vi "Keithley 6514 Buffer Read.vi"(0 "Resource In":refnum<visa-resource-name>, 1 "Check For SCPI Errors? (T)":bool=TRUE, 11 "error in (no error)":T1) -> (4 "Resource Out (dupl)":refnum<visa-resource-name>, 6 "Num Readings":i32 min=0 max=2500, 8 "Test Data":sgl[][](array[numeric]) format="%^.4e", 10 "Data Elements":string, 15 "error out":T1)   [LabVIEW 2009, in "Keithley 6514 LV 2009.lvlib"]
doc: "This VI is used to retrieve data from the Instrument's data buffer. The VI will return the number of points that was stored in the buffer, the data format used for the data transfer, the data elements returned and the actual data which is stored in a LabVIEW array.\n\nDEFAULTS: \nGPIB Address = 7\n\nPoints Stored in Buffer:\nReturned by Instrument. Not user settable. 2 to 1024.\n\nData Format: \nReturned by Instrument. Not user settable. Format returned is 'ASC' for ASCII and 'SRE' for Single Precision Real.\n\nData Elements:\nReturned by Instrument. Not user settable. The order in which the elements are returned reflects the order in which each data point is presented in the array. Main order is:\nReading, Channel Number\n\nTest Data:\nThis is an array where the buffer data is placed after transfer over the bus. The order for which the data is presented appears in the 'Data Elements' indicator. Maximum number of data points returned is 1024."
uses:
  Keithley 6514 LV 2009.lvlib
panel:
  in  "Timeout (5000 msecs)":u32=5000
  out "Num Bytes To Read For Binary":i32
  out "Data Format":string
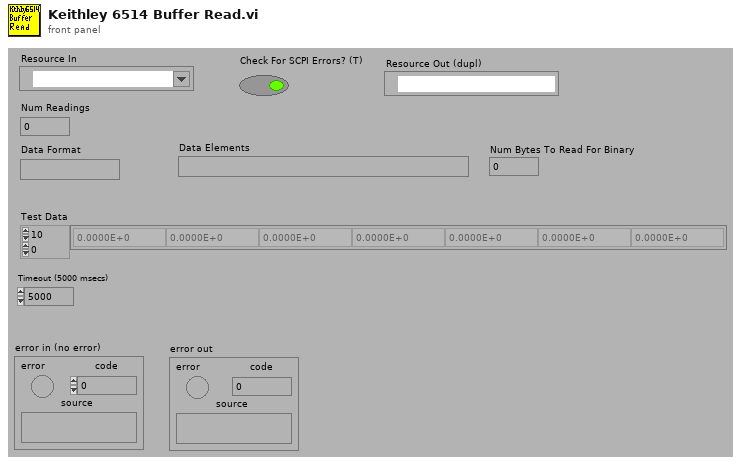
[diagram p1: front panel]
types:
  T1 = cluster{"error":bool, "code":i32, "source":string}
  T2 = enum16{"big-endian, network order", "native, host order", "little-endian"}
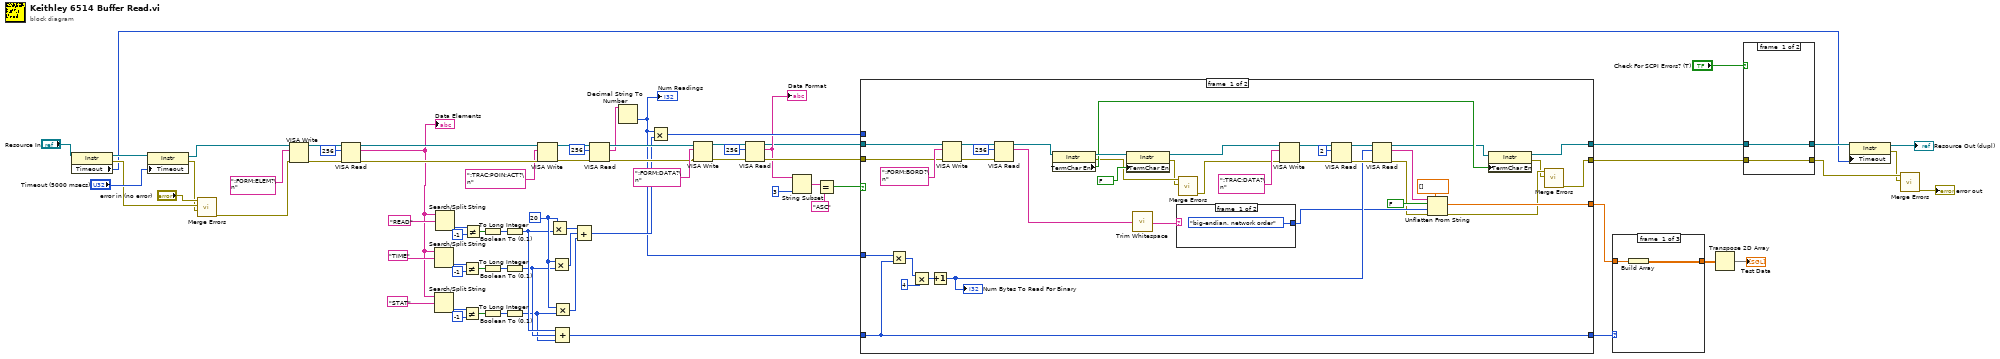
[diagram p0: block diagram]
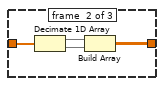
[diagram p2: hidden frame]
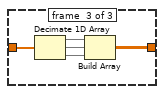
[diagram p3: hidden frame]
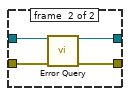
[diagram p4: hidden frame]
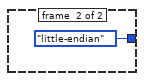
[diagram p5: hidden frame]
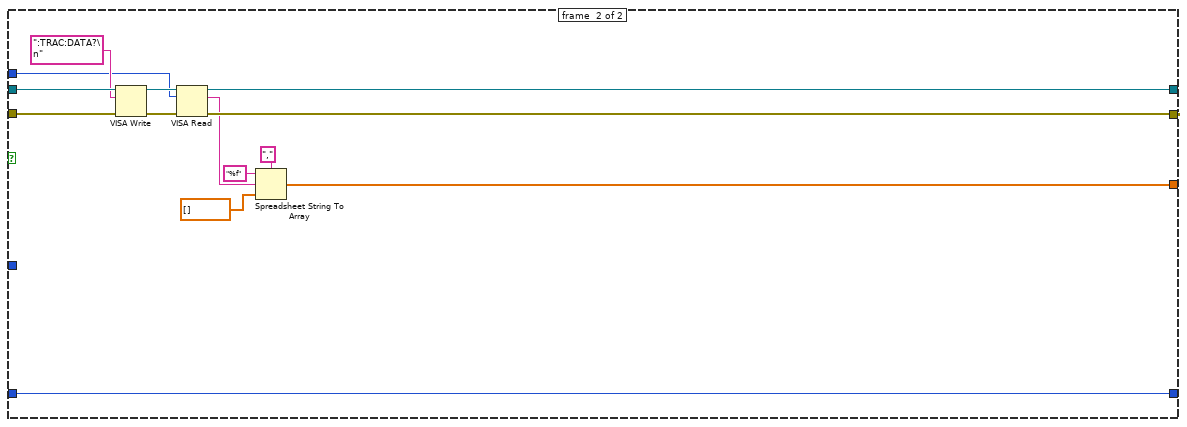
[diagram p6: hidden frame]
diagram:
  w28 = 20 ("x")
  n1 = property class="Instr"(reference="Resource In") -> (reference out=w12:refnum<visa-resource-name>, error out=w10:errorcluster, "Timeout"=w4:u32)  [unwired: 1 in]
  n2 = property class="Instr"(reference=w12, "Timeout"="Timeout (5000 msecs)") -> (reference out=w7:refnum<visa-resource-name>, error out=w9:errorcluster)  [unwired: 1 in]
  n3 = call <vilib>:"Merge Errors.vi"("error in 3 (no error)"=w9, "error in 2 (no error)"=w10, "error in 1 (no error)"="error in (no error)") -> ("error out"=w8:errorcluster)  [unwired: 4 in]
  n4 = VISA Write(VISA resource name=w7, write buffer=":FORM:ELEM?\n", error in (no error)=w8) -> (VISA resource name out=w65:refnum<visa-resource-name>, error out=w64:errorcluster)  [unwired: 1 out]
  n5 = VISA Read(VISA resource name=w65, byte count=u32 256, error in (no error)=w64) -> (VISA resource name out=w58:refnum<visa-resource-name>, read buffer=w36:string, error out=w59:errorcluster)  [unwired: 1 out]
  "Data Elements" <- w36
  n6 = Search/Split String(string=w36, search string/char (-)="TIME") -> (offset of match=w41:i32)  [unwired: 1 in, 2 out]
  n7 = Search/Split String(string=w36, search string/char (-)="STAT") -> (offset of match=w38:i32)  [unwired: 1 in, 2 out]
  n8 = Search/Split String(string=w36, search string/char (-)="READ") -> (offset of match=w43:i32)  [unwired: 1 in, 2 out]
  n9 = Not Equal?(x=w41, y=-1) -> (x != y?=w33:bool)
  n10 = Not Equal?(x=w38, y=-1) -> (x != y?=w32:bool)
  n11 = Not Equal?(x=w43, y=-1) -> (x != y?=w34:bool)
  n12 = Boolean To (0,1)(Boolean=w34) -> (0, 1=w31:i16)
  n13 = Boolean To (0,1)(Boolean=w33) -> (0, 1=w30:i16)
  n14 = Boolean To (0,1)(Boolean=w32) -> (0, 1=w29:i16)
  n15 = To Long Integer(number=w31) -> (32bit integer=w23:i32)
  n16 = To Long Integer(number=w30) -> (32bit integer=w22:i32)
  n17 = To Long Integer(number=w29) -> (32bit integer=w21:i32)
  n18 = VISA Write(VISA resource name=w58, write buffer=":TRAC:POIN:ACT?\n", error in (no error)=w59) -> (VISA resource name out=w61:refnum<visa-resource-name>, error out=w60:errorcluster)  [unwired: 1 out]
  n19 = Multiply(x=w28, y=w23) -> (x*y=w27:i32)
  n20 = Multiply(x=w28, y=w22) -> (x*y=w26:i32)
  n21 = Multiply(x=w28, y=w21) -> (x*y=w25:i32)
  n22 = Compound Arithmetic op=ADD(w23, w22, w21) -> (w20:i32)
  n23 = Compound Arithmetic op=ADD(w27, w26, w25) -> (w24:i32)
  n24 = VISA Read(VISA resource name=w61, byte count=u32 256, error in (no error)=w60) -> (VISA resource name out=w52:refnum<visa-resource-name>, read buffer=w50:string, error out=w51:errorcluster)  [unwired: 1 out]
  n25 = Decimal String To Number(string=w50) -> (number=w19:i32)  [unwired: 2 in, 1 out]
  "Num Readings" <- w19
  n26 = Multiply(x=w19, y=w24) -> (x*y=w68:i32)
  n27 = VISA Write(VISA resource name=w52, write buffer=":FORM:DATA?\n", error in (no error)=w51) -> (VISA resource name out=w55:refnum<visa-resource-name>, error out=w54:errorcluster)  [unwired: 1 out]
  n28 = VISA Read(VISA resource name=w55, byte count=u32 256, error in (no error)=w54) -> (VISA resource name out=w47:refnum<visa-resource-name>, read buffer=w48:string, error out=w49:errorcluster)  [unwired: 1 out]
  "Data Format" <- w48
  n29 = String Subset(string=w48, length (rest)=3) -> (substring=w70:string)  [unwired: 1 in]
  n30 = Equal?(x=w70, y="ASC") -> (x = y?=w69:bool)
  n31 = case shown="False" w69 {
    tunnel: w49 -> [w90 w126]
    tunnel: w68 -> [_ w120]
    tunnel: w20 -> [w79 w114]
    tunnel: w19 -> [w109 _]
    tunnel: [w73 w127] -> w44
    tunnel: w47 -> [w91 w125]
    tunnel: [w96 w121] -> w45
    tunnel: [w80 w115] -> w17
    tunnel: [w79 w114] -> w18
    frame #0 {
      n32 = Multiply(x=w109, y=w79) -> (x*y=w111:i32)
      n33 = Multiply(x=w111, y=4) -> (x*y=w108:i32)
      n34 = Increment(x=w108) -> (x+1=w89:i32)
      "Num Bytes To Read For Binary" <- w89
      n35 = VISA Write(VISA resource name=w91, write buffer=":FORM:BORD?\n", error in (no error)=w90) -> (VISA resource name out=w94:refnum<visa-resource-name>, error out=w93:errorcluster)  [unwired: 1 out]
      n36 = VISA Read(VISA resource name=w94, byte count=u32 256, error in (no error)=w93) -> (VISA resource name out=w88:refnum<visa-resource-name>, read buffer=w85:string)  [unwired: 2 out]
      n37 = property class="Instr"(reference=w88) -> (reference out=w107:refnum<visa-resource-name>, error out=w76:errorcluster, "TermChar En"=w97:bool)  [unwired: 1 in]
      n38 = property class="Instr"(reference=w107, "TermChar En"=FALSE ("Message Based Settings:Termination Character Enable")) -> (reference out=w102:refnum<visa-resource-name>, error out=w75:errorcluster)  [unwired: 1 in]
      n39 = call <vilib>:"Trim Whitespace.vi"("string"=w85) -> ("trimmed string"=w82:string)  [unwired: 1 in]
      n40 = case shown="\"SWAP\"" w82 {
        tunnel: [T2."big-endian, network order" ("byte order (0:big-endian, network order)") T2."little-endian" ("byte order (0:big-endian, network order)")] -> w84
        frame #0 {
        }
        frame #1 {
        }
      }
      n41 = call <vilib>:"Merge Errors.vi"("error in 2 (no error)"=w75, "error in 1 (no error)"=w76) -> ("error out"=w78:errorcluster)  [unwired: 5 in]
      n42 = VISA Write(VISA resource name=w102, write buffer=":TRAC:DATA?\n", error in (no error)=w78) -> (VISA resource name out=w104:refnum<visa-resource-name>, error out=w103:errorcluster)  [unwired: 1 out]
      n43 = VISA Read(VISA resource name=w104, byte count=u32 2, error in (no error)=w103) -> (VISA resource name out=w99:refnum<visa-resource-name>, error out=w100:errorcluster)  [unwired: 2 out]
      n44 = VISA Read(VISA resource name=w99, byte count=w89, error in (no error)=w100) -> (VISA resource name out=w81:refnum<visa-resource-name>, read buffer=w87:string, error out=w83:errorcluster)  [unwired: 1 out]
      n45 = Unflatten From String(type=sgl[] [], binary string=w87, data includes array or string size? (T)=FALSE, byte order (0:big-endian, network order)=w84, error in (no error)=w83) -> (value=w80:sgl[], error out=w77:errorcluster)  [unwired: 1 out]
      n46 = property class="Instr"(reference=w81, "TermChar En"=w97) -> (reference out=w96:refnum<visa-resource-name>, error out=w74:errorcluster)  [unwired: 1 in]
      n47 = call <vilib>:"Merge Errors.vi"("error in 2 (no error)"=w74, "error in 1 (no error)"=w77) -> ("error out"=w73:errorcluster)  [unwired: 5 in]
    }
    frame #1 {
      n48 = VISA Write(VISA resource name=w125, write buffer=":TRAC:DATA?\n", error in (no error)=w126) -> (VISA resource name out=w122:refnum<visa-resource-name>, error out=w123:errorcluster)  [unwired: 1 out]
      n49 = VISA Read(VISA resource name=w122, byte count=w120, error in (no error)=w123) -> (VISA resource name out=w121:refnum<visa-resource-name>, read buffer=w119:string, error out=w127:errorcluster)  [unwired: 1 out]
      n50 = Spreadsheet String To Array(delimiter (Tab)=",", format string="%f", spreadsheet string=w119, array type (2D Dbl)=sgl[] []) -> (array=w115:sgl[])
    }
  }
  n51 = case shown="Default" w18 {
    tunnel: [w128 w130 w134] -> w16
    tunnel: w17 -> [w129 w133 w138]
    frame #0 {
      n52 = Build Array(w129) -> (w128:sgl[][])
    }
    frame #1 {
      n53 = Decimate 1D Array(w133) -> (w132:sgl[], w131:sgl[])
      n54 = Build Array(w132, w131) -> (w130:sgl[][])
    }
    frame #2 {
      n55 = Decimate 1D Array(w138) -> (w137:sgl[], w136:sgl[], w135:sgl[])
      n56 = Build Array(w137, w136, w135) -> (w134:sgl[][])
    }
  }
  n57 = Transpose 2D Array(2D array=w16) -> (transposed array=→"Test Data":sgl[][])
  n58 = case shown="False" "Check For SCPI Errors? (T)" {
    tunnel: w45 -> [w140 w144]
    tunnel: w44 -> [w139 w143]
    tunnel: [w140 w142] -> w6
    tunnel: [w139 w141] -> w3
    frame #0 {
    }
    frame #1 {
      n59 = call "Error Query.vi"("VISA Resource In"=w144, "error in (no error)"=w143) -> ("VISA Resource Out (dupl)"=w142:refnum<visa-resource-name>, "error out"=w141:errorcluster)  [unwired: 10 in, 2 out]
    }
  }
  n60 = property class="Instr"(reference=w6, "Timeout"=w4) -> (reference out=→"Resource Out (dupl)":refnum<visa-resource-name>, error out=w2:errorcluster)  [unwired: 1 in]
  n61 = call <vilib>:"Merge Errors.vi"("error in 2 (no error)"=w2, "error in 1 (no error)"=w3) -> ("error out"=→"error out":errorcluster)  [unwired: 5 in]
